vi "Digital Write 1 channel.vi"(8 "error in (no error)":errorcluster, 9 "On/Off":bool, 10 "Channel":i32, 11 "Initial State":bool[](array[boolean])) -> (0 "error out":errorcluster, 3 "FinalState":bool[](array[boolean]))   [LabVIEW 2016]
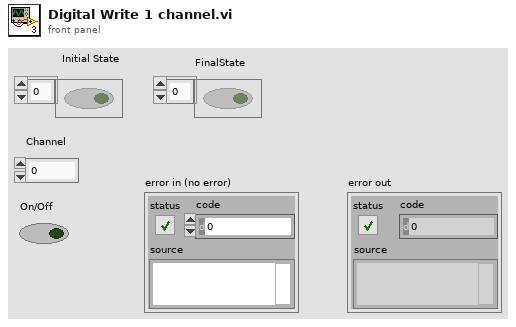
[diagram p1: front panel]
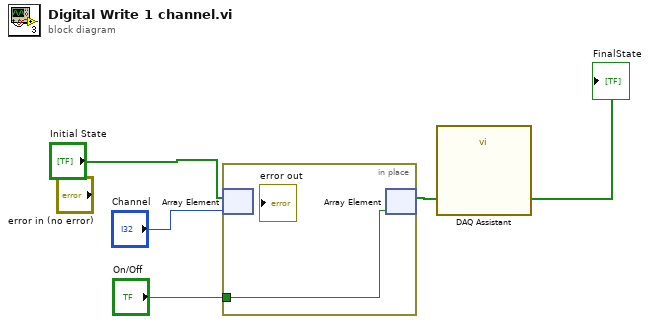
[diagram p0: block diagram]
diagram:
  n1 = in-place {
    in-place-border: "On/Off" -> [w5]
    n2 = in-place-array #1("Initial State", "Channel") -> ()  [unwired: 1 out]
    n3 = in-place-array #1(w5) -> (w4:bool[])  [unwired: 1 out]
  }
  "FinalState" <- w4
  n4 = call "DAQ Assistant"("data"=w4) -> ()  [unwired: 17 in, 2 out]
